vi "SeqnSetElectd.vi"(6 "Group #":u8, 7 "Amplitude":sgl, 8 "Index":u8, 9 "Electrode Ref":refnum<vi>) -> ()   [LabVIEW 2012, in "Sequence.lvclass"]
uses:
  Sequence.lvclass
  UserControl/ElectdPanel.ctl
  UserControl/ElectdTerminal.ctl
  StimulCtrls.lvlib
panel:
  in  "Terminal":u8(ring)
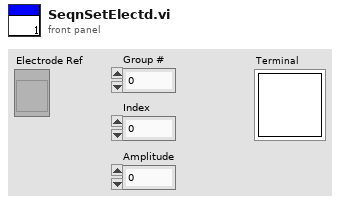
[diagram p1: front panel]
types:
  T1 = enum8{"Enabled", "Disabled", "Disabled and Grayed Out"}
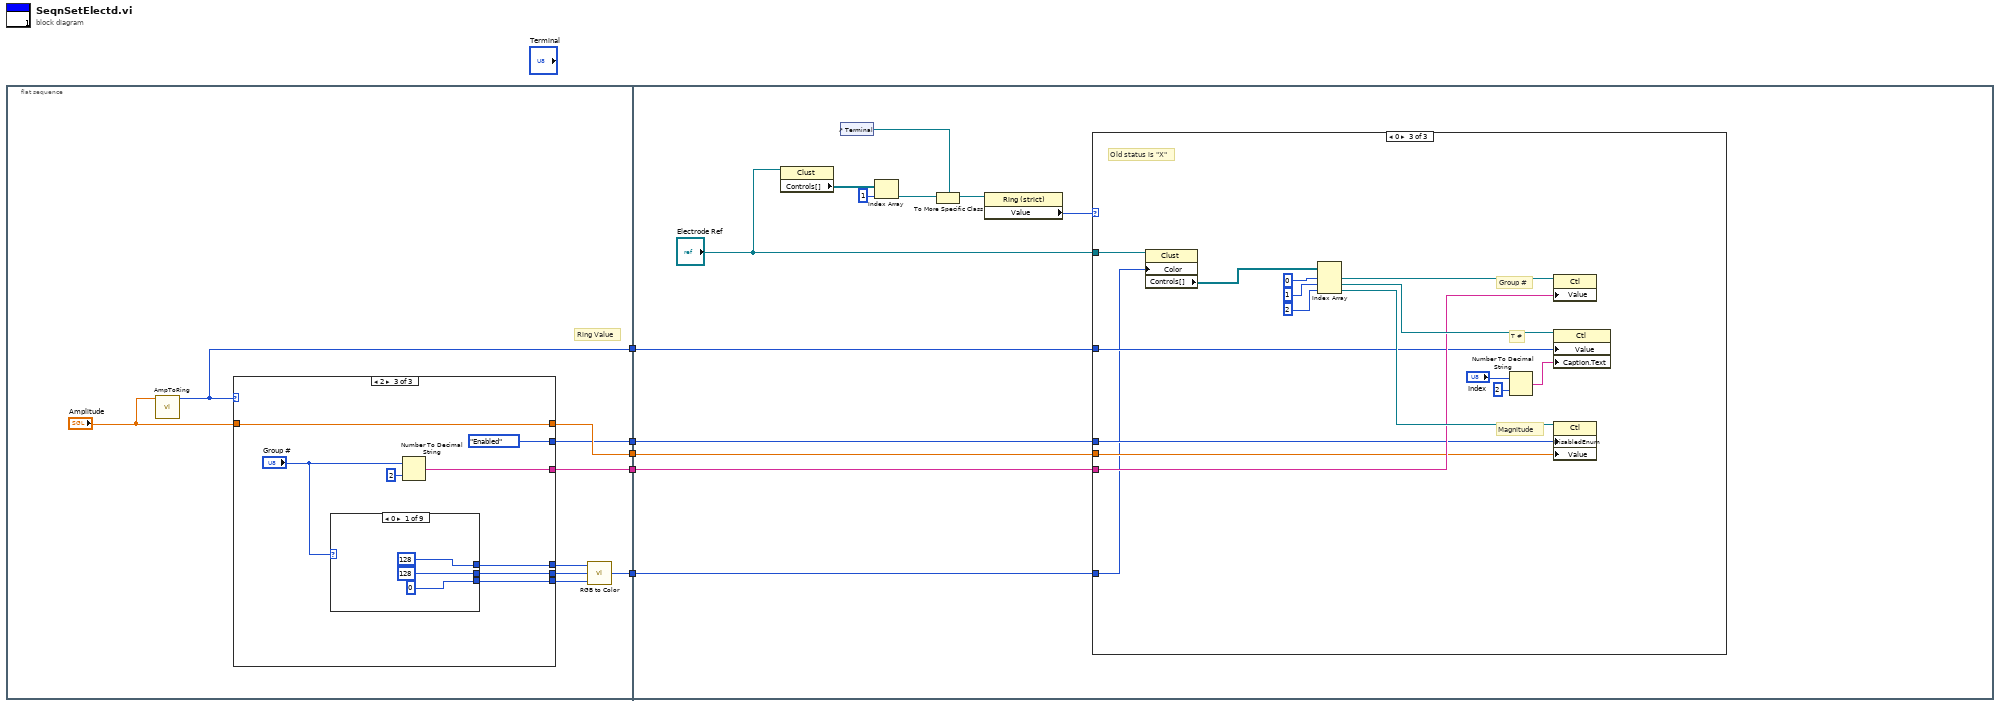
[diagram p0: block diagram]
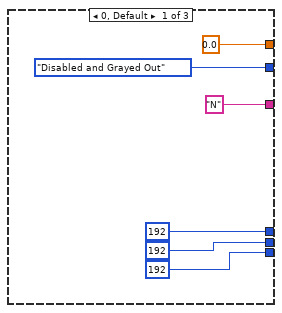
[diagram p2: hidden frame]
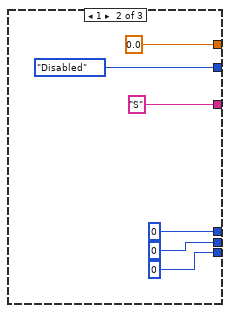
[diagram p3: hidden frame]
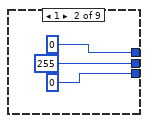
[diagram p4: hidden frame]
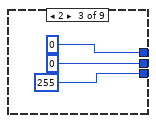
[diagram p5: hidden frame]
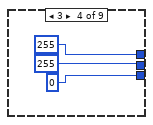
[diagram p6: hidden frame]
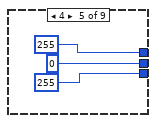
[diagram p7: hidden frame]
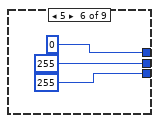
[diagram p8: hidden frame]
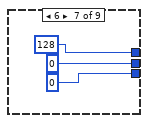
[diagram p9: hidden frame]
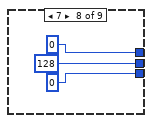
[diagram p10: hidden frame]
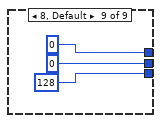
[diagram p11: hidden frame]
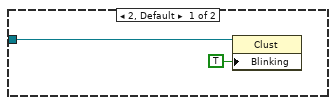
[diagram p13: hidden frame]
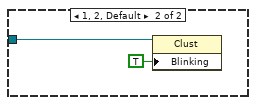
[diagram p15: hidden frame]
diagram:
  n1 = flat-sequence {
    tunnel: [w10] -> w5
    tunnel: [w9] -> w4
    tunnel: [w8] -> w3
    tunnel: [w7] -> w2
    tunnel: [w6] -> w1
    tunnel: w5 -> [w62]
    tunnel: w4 -> [w73]
    tunnel: w3 -> [w71]
    tunnel: w2 -> [w72]
    tunnel: w1 -> [w70]
    frame #0 {
      # "Ring Value"
      n2 = call "AmpToRing.vi"("Amplitude"="Amplitude") -> ("Ring Value"=w6:u8)  [unwired: 10 in]
      n3 = case shown="2" w6 {
        tunnel: ["N" ("Group #") "S" ("Group #") w28] -> w9
        tunnel: [T1."Disabled and Grayed Out" ("Disabled") T1."Disabled" ("Disabled") T1."Enabled" ("Disabled")] -> w7
        tunnel: [u32 192 ("Color") u32 0 ("Color") w33] -> w11
        tunnel: [u32 192 ("Color") u32 0 ("Color") w32] -> w12
        tunnel: [u32 192 ("Color") u32 0 ("Color") w31] -> w13
        tunnel: "Amplitude" -> [_ _ w29]
        tunnel: [sgl 0.0 ("Magnitude") sgl 0.0 ("Magnitude") w29] -> w8
        frame 0, Default {
        }
        frame 1 {
        }
        frame 2 {
          n4 = case shown="0" "Group #" {
            tunnel: [u32 128 ("Color") u32 0 ("Color") u32 0 ("Color") u32 255 ("Color") u32 255 ("Color") u32 0 ("Color") u32 128 ("Color") u32 0 ("Color") u32 0 ("Color")] -> w33
            tunnel: [u32 128 ("Color") u32 255 ("Color") u32 0 ("Color") u32 255 ("Color") u32 0 ("Color") u32 255 ("Color") u32 0 ("Color") u32 128 ("Color") u32 0 ("Color")] -> w32
            tunnel: [u32 0 ("Color") u32 0 ("Color") u32 255 ("Color") u32 0 ("Color") u32 255 ("Color") u32 255 ("Color") u32 0 ("Color") u32 0 ("Color") u32 128 ("Color")] -> w31
            frame 0 {
            }
            frame 1 {
            }
            frame 2 {
            }
            frame 3 {
            }
            frame 4 {
            }
            frame 5 {
            }
            frame 6 {
            }
            frame 7 {
            }
            frame 8, Default {
            }
          }
          n5 = Number To Decimal String(number="Group #", width (-)=i16 2) -> (decimal integer string=w28:string)
        }
      }
      n6 = call <vilib>:"RGB to Color.vi"("B"=w13, "G"=w12, "R"=w11) -> ("Color"=w10:u32)
    }
    frame #1 {
      n7 = property class="Clust"(reference="Electrode Ref") -> ("Controls[]"=w68:refnum<vi>[])  [unwired: 1 in, 2 out]
      n8 = control-ref of="Terminal"() -> (w63:refnum<vi>)
      n9 = Index Array(array=w68, index=1) -> (element=w66:refnum<vi>)
      n10 = To More Specific Class(target class=w63, reference=w66) -> (specific class reference=w65:refnum<vi>)  [unwired: 1 in, 1 out]
      n11 = property class="Ring (strict)"(reference=w65) -> ("Value"=w64:u8)  [unwired: 1 in, 2 out]
      n12 = case shown="0" w64 {
        tunnel: w73 -> [_ _ w88]
        tunnel: w72 -> [_ _ w87]
        tunnel: w71 -> [_ _ w86]
        tunnel: w70 -> [w75 w78 w85]
        tunnel: "Electrode Ref" -> [w74 w79 w84]
        tunnel: w62 -> [_ _ w83]
        frame 1 {
          # "Old status is \"+\""
          n13 = case shown="0, 1" w75 {
            tunnel: w74 -> [w77 _]
            frame 2, Default {
              n14 = property class="Clust"(reference=w77, "Blinking"=TRUE) -> ()  [unwired: 1 in, 2 out]
            }
            frame 0, 1 {
            }
          }
        }
        frame 2, Default {
          # "Old status is \"-\""
          n15 = case shown="0" w78 {
            tunnel: w79 -> [_ w80]
            frame 0 {
            }
            frame 1, 2, Default {
              n16 = property class="Clust"(reference=w80, "Blinking"=TRUE) -> ()  [unwired: 1 in, 2 out]
            }
          }
        }
        frame 0 {
          # "Old status is \"X\""
          # "Group #"
          # "Magnitude"
          # "T #"
          n17 = property class="Clust"(reference=w84, "Color"=w83) -> ("Controls[]"=w82:refnum<vi>[])  [unwired: 1 in, 2 out]
          n18 = Index Array(array=w82, index #1=0 ("index"), index #2=1 ("index"), index #3=2 ("index")) -> (element #1=w97:refnum<vi>, element #2=w96:refnum<vi>, element #3=w95:refnum<vi>)
          n19 = Number To Decimal String(number="Index", width (-)=i16 2) -> (decimal integer string=w94:string)
          n20 = property class="Ctl"(reference=w97, "Value"=w88) -> ()  [unwired: 1 in, 2 out]
          n21 = property class="Ctl"(reference=w96, "Value"=w85, "Caption.Text"=w94) -> ()  [unwired: 1 in, 2 out]
          n22 = property class="Ctl"(reference=w95, "DisabledEnum"=w87, "Value"=w86) -> ()  [unwired: 1 in, 2 out]
        }
      }
    }
  }
